vi "Transmitter_SC - Optimized.vi"() -> ()   [LabVIEW 2022 SP3]
uses:
  <instrlib>/niUSRP/niUSRP Write Tx Data (CDB Cluster).vi
panel:
  in  "Alpha":dbl(slide)=0.17500000000000002 step=0.005 scale=0.0..1.0
  in  "Tab Control":enum32{"USRP Parameters", "Transmission"}(tab)
  in  "USRP ControledParameters 2":T1={"Active Antenna"="TX1", "Gain (dB)"=0.0, "Carrier Frequency"=2400000000.0, "IQ Rate"=2000000.0, "Active Channel"="0"} {"IQ Rate" format="%#_6p"; "Carrier Frequency" format="%#_6p"; "Gain (dB)" format="%#_6f"}
  in  "Device selection":refnum<k15>="RIO0"
  in  "stop":bool
  out "Error out":errorcluster
  in  "Modulation parameter":T2
  out "Bits length":i32
  out "Bits length 2":i32
  out "Frame Duration":dbl format="%#_6p"
  out "Coerced Parameters":T3={"IQ Rate"=100000.0, "Carrier  Freq."=100000.0, "Gain"=0.0} {"Gain" format="%#_6f"; "Carrier  Freq." format="%#_6p"; "IQ Rate" format="%#_6p"}
  out "Transmitted Waveform":cluster{"t0":dbl, "dt":dbl, "Y":dbl[]}(graph)
  in  "Message 2":string="ptua. At vero eos et accusam et justo duo dolores et ea rebum. Stet clita kasd gubergren, no sea takimata sanctus est Lorem ipsum dolor sit amet. Lore"
  in  "Message 1":string="Lorem ipsum dolor sit amet, consetetur sadipscing elitr, sed diam nonumy eirmod tempor invidunt ut labore et dolore magna aliquyam erat, sed diam volu"
  in  "error in (no error)":errorcluster
  # "OFDM Superposition Coded Transmitter"
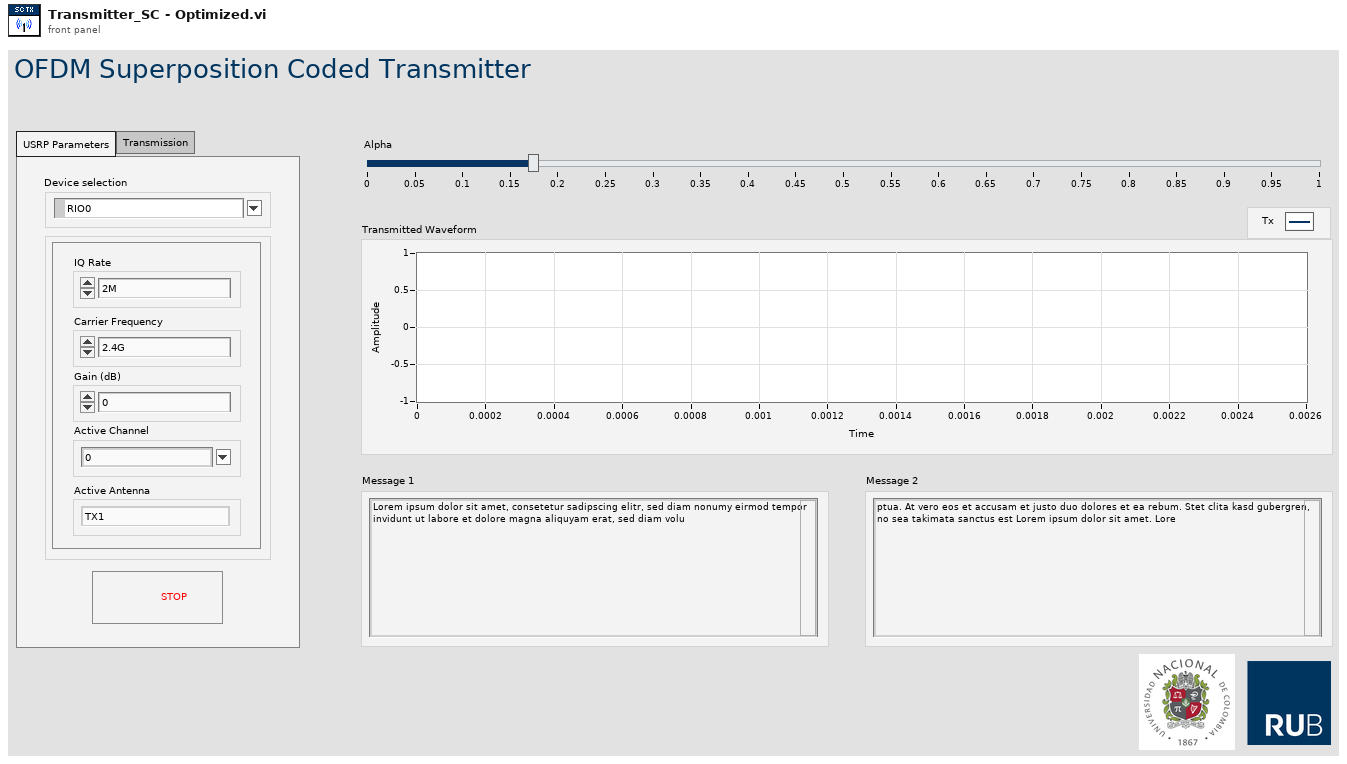
[diagram p1: front panel]
types:
  T1 = cluster{"Active Antenna":string, "Gain (dB)":dbl, "Carrier Frequency":dbl, "IQ Rate":dbl, "Active Channel":string}
  T2 = cluster{"Modulation type":enum16{"QPSK(4QAM)", "64QAM", "16QAM", "BPSK"}, "BCC rate (k/n)":enum16{"1/2", "2/3", "3/4"}}
  T3 = cluster{"IQ Rate":dbl, "Carrier  Freq.":dbl, "Gain":dbl}
  T4 = cluster{"coerced IQ rate":dbl, "coerced carrier frequency":dbl, "coerced gain":dbl}
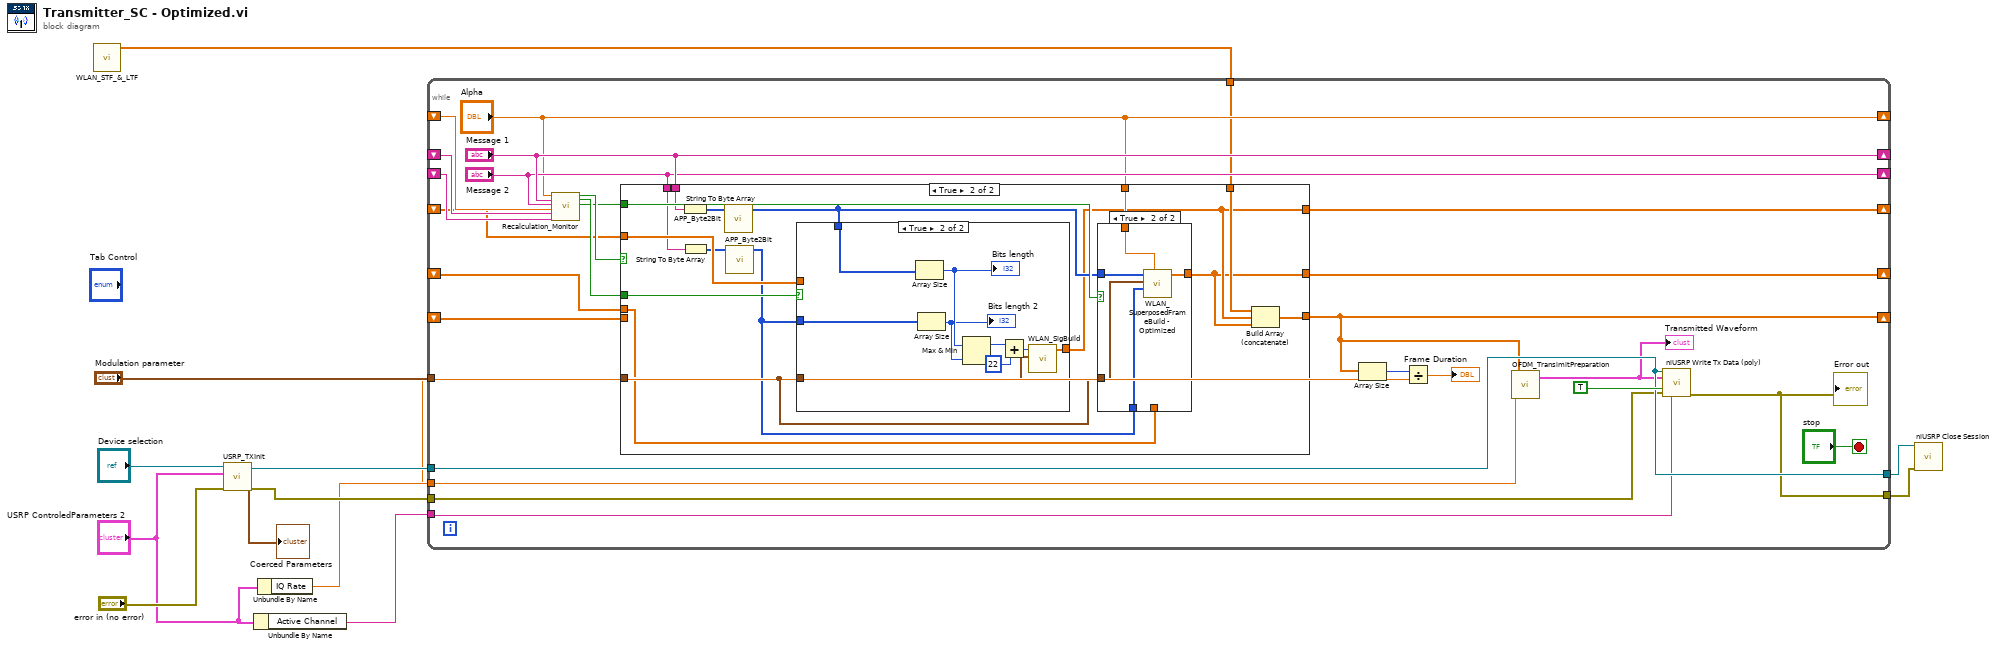
[diagram p0: block diagram]
diagram:
  n1 = call "WLAN_STF_&_LTF.vi"() -> ("STF & LTF"=w1:cdb[])  [unwired: 11 in]
  n2 = call "USRP_TXInit.vi"("device names"="Device selection", "USRP ControledParameters"="USRP ControledParameters 2", "error in (no error)"="error in (no error)") -> ("session handle out"=w11:refnum<k15>, "USRP CoercedParamters"=→"Coerced Parameters":T4, "error out"=w10:errorcluster)  [unwired: 5 in]
  n3 = Unbundle By Name("USRP ControledParameters 2") -> ("Active Channel"=w3:string)
  n4 = Unbundle By Name("USRP ControledParameters 2") -> ("IQ Rate"=w9:dbl)
  n5 = while {
    tunnel: w11 -> [w35]
    tunnel: w10 -> [w13]
    tunnel: w9 -> [w34]
    tunnel: [w35] -> w8
    tunnel: [w32] -> w7
    tunnel: w3 -> [w31]
    shift-right: ["Alpha"] -> _
    shift-left: _ -> [w30]
    shift-right: ["Message 1"] -> _
    shift-left: _ -> [w29]
    shift-right: ["Message 2"] -> _
    shift-left: _ -> [w28]
    tunnel: "Modulation parameter" -> [w22]
    shift-right: [w21] -> _
    shift-left: _ -> [w20]
    shift-right: [w18] -> _
    shift-left: _ -> [w17]
    tunnel: w1 -> [w16]
    shift-right: [w14] -> _
    shift-left: _ -> [w15]
    stop <- "stop" stop-if-true
    n6 = call "Recalculation_Monitor.vi"("Alpha"="Alpha", "Message 1"="Message 1", "Message 2"="Message 2", "Alpha old"=w30, "Message 1 old"=w29, "Message 2 old"=w28) -> ("Recalculate?"=w27:bool, "Recalculate SIG"=w26:bool, "Recalculate OFDM"=w25:bool)  [unwired: 11 in]
    n7 = case shown="True" w27 {
      tunnel: w26 -> [_ w58]
      tunnel: w25 -> [_ w57]
      tunnel: "Message 1" -> [_ w52]
      tunnel: "Message 2" -> [_ w53]
      tunnel: w22 -> [_ w49]
      tunnel: [w42 w45] -> w21
      tunnel: w20 -> [w42 w56]
      tunnel: "Alpha" -> [_ w48]
      tunnel: [w41 w44] -> w18
      tunnel: w17 -> [w41 w47]
      tunnel: w16 -> [_ w46]
      tunnel: [w40 w43] -> w14
      tunnel: w15 -> [w40 _]
      frame False {
      }
      frame True {
        n8 = String To Byte Array(string=w52) -> (unsigned byte array=w54:u8[])
        n9 = String To Byte Array(string=w53) -> (unsigned byte array=w55:u8[])
        n10 = call "APP_Byte2Bit.vi"("input byte stream"=w54) -> ("output bit stream"=w50:i8[])  [unwired: 10 in]
        n11 = call "APP_Byte2Bit.vi"("input byte stream"=w55) -> ("output bit stream"=w51:i8[])  [unwired: 10 in]
        n12 = case shown="True" w58 {
          tunnel: w49 -> [_ w66]
          tunnel: [w65 w72] -> w45
          tunnel: w56 -> [w65 _]
          tunnel: w51 -> [_ w68]
          tunnel: w50 -> [_ w67]
          frame False {
          }
          frame True {
            n13 = Array Size(array=w67) -> (size(s)=w74:i32)
            "Bits length" <- w74
            n14 = Array Size(array=w68) -> (size(s)=w73:i32)
            "Bits length 2" <- w73
            n15 = Max & Min(x=w74, y=w73) -> (max(x,y)=w70:i32)  [unwired: 1 out]
            n16 = Add(x=w70, y=22) -> (x+y=w71:i32)
            n17 = call "WLAN_SigBuild.vi"("Data bit length"=w71, "Modulation parameter"=w66) -> ("symbols"=w72:cdb[])  [unwired: 7 in, 1 out]
          }
        }
        n18 = case shown="True" w57 {
          tunnel: w51 -> [_ w64]
          tunnel: w50 -> [_ w63]
          tunnel: w49 -> [_ w62]
          tunnel: w48 -> [_ w61]
          tunnel: [w59 w60] -> w44
          tunnel: w47 -> [w59 _]
          frame False {
          }
          frame True {
            n19 = call "WLAN_SuperposedFrameBuild - Optimized.vi"("Alpha"=w61, "data in 2"=w64, "Modulation parameter"=w62, "data in"=w63) -> ("output array"=w60:cdb[])  [unwired: 6 in, 1 out]
          }
        }
        n20 = Build Array (concatenate)(w46, w45, w44) -> (w43:cdb[])
      }
    }
    n21 = Array Size(array=w14) -> (size(s)=w37:i32)
    n22 = Divide(x=w37, y=w34) -> (x/y=→"Frame Duration":dbl)
    n23 = call "OFDM_TransimitPreparation.vi"("IQ rate"=w34, "array"=w14) -> ("output cluster"=w33:cluster{"t0":dbl, "dt":dbl, "Y":cdb[]})  [unwired: 9 in]
    "Transmitted Waveform" <- w33
    n24 = call-poly <instrlib>:"niUSRP Write Tx Data (poly).vi"("session handle"=w35, "channel list"=w31, "data"=w33, "end of data?"=TRUE, "error in (no error)"=w13) -> ("error out"=w32:errorcluster)  [unwired: 9 in, 1 out]
    "Error out" <- w32
  }
  n25 = call <instrlib>:"niUSRP Close Session.vi"("session handle"=w8, "error in (no error)"=w7) -> ()  [unwired: 13 in, 1 out]
